vi "Register Read.vi"(0 "instrument handle in":refnum<k15>, 1 "Bus Number":i32, 5 "Slave Address":T3=12 format="%02x", 7 "Register Address":T2 format="%02x", 11 "error in (no error)":errorcluster) -> (4 "instrument handle out":refnum<k15>, 6 "Register Data":T1 format="%02x", 15 "error out":errorcluster)   [LabVIEW 2018, in "MIPI RFFE API.lvlib"]
uses:
  MIPI RFFE API.lvlib
  Slave Address.ctl
  Register Address.ctl
  Register Data.ctl
  Standard Command/RFFE Standard Command.lvclass/RFFE Standard Command.ctl
  Standard Command/Get Register Data.vi
  RegRead/RFFE RegRead Command.lvclass
  C:/Users/semoore/Projects/mipi-rffe-labview-oop/Standard Command/RFFE Standard Command.lvclass
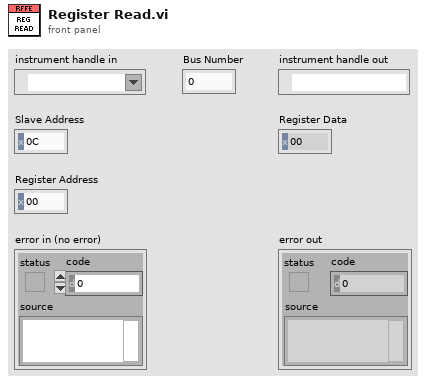
[diagram p1: front panel]
types:
  T1 = typedef "MIPI RFFE API.lvlib/Register Data.ctl" = u8
  T2 = typedef "MIPI RFFE API.lvlib/Register Address.ctl" = u16
  T3 = typedef "MIPI RFFE API.lvlib/Slave Address.ctl" = u8
  T4 = typedef "RFFE Commands.lvlib/Register Data.ctl" = u8
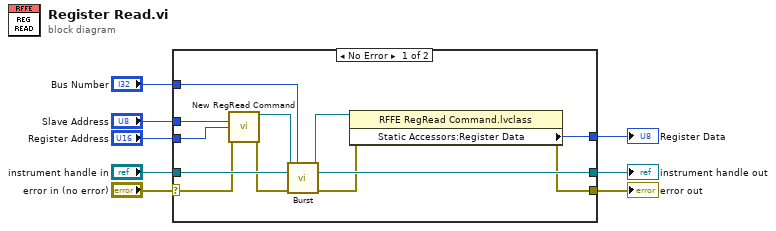
[diagram p0: block diagram]
diagram:
  n1 = case shown="No Error" "error in (no error)" {
    selector: "error in (no error)" -> [w18 w21]
    tunnel: "instrument handle in" -> [w20 w22]
    tunnel: [w19 w22] -> w7
    tunnel: "Slave Address" -> [w16 _]
    tunnel: "Register Address" -> [w15 _]
    tunnel: [w11 w21] -> w3
    tunnel: [w10 _] -> w2
    tunnel: "Bus Number" -> [w9 _]
    frame No Error {
      n2 = call "New RegRead Command.vi"("Slave Address"=w16, "Register Address"=w15, "error in (no error)"=w18) -> ("RFFE RegRead Command out"=w14:refnum<class "RFFE RegRead Command.lvclass">, "error out"=w17:errorcluster)  [unwired: 11 in]
      n3 = call-dynamic "Burst.vi"("RFFE RegRead Command in"=w14, "Bus Number"=w9, "instrument handle in"=w20, "error in (no error)"=w17) -> ("RFFE RegRead Command out"=w13:refnum<class "RFFE RegRead Command.lvclass">, "instrument handle out"=w19:refnum<k15>, "error out"=w12:errorcluster)  [unwired: 9 in]
      n4 = property class="RFFE RegRead Command.lvclass"(reference=w13, error in=w12) -> (error out=w11:errorcluster, "Static Accessors:Register Data"=w10:T4)  [unwired: 1 out]
    }
    frame Error {
    }
  }
  "instrument handle out" <- w7
  "error out" <- w3
  "Register Data" <- w2
